vi "ConfigureDlg.vi"(8 "error in (no error)":errorcluster, 11 "Local in":refnum<class "Local.lvclass">) -> (0 "error out":errorcluster, 2 "Changed?":bool, 3 "Local out":refnum<class "Local.lvclass">)   [LabVIEW 2014, in "SyncPlugins.lvlib" / "Local.lvclass"]
uses:
  Local.lvclass
panel:
  in  "btnDone":bool
  # "Local Sync Module has no configurable Parameters"
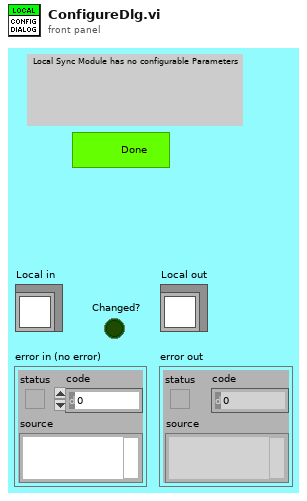
[diagram p1: front panel]
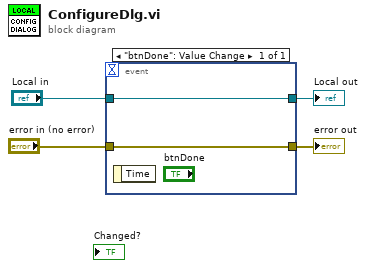
[diagram p0: block diagram]
diagram:
  n1 = event shown="[0] \"btnDone\": Value Change" {
    selector: _ -> [_]
    dyn-events: _ -> [_]
    timeout: _ -> [_]
    tunnel: "error in (no error)" -> [w6]
    tunnel: [w6] -> w3
    tunnel: [w5] -> w1
    tunnel: "Local in" -> [w5]
    event "btnDone": Value Change {
      n2 = event-data() -> ()  [unwired: 1 in, 1 out]
    }
  }
  "error out" <- w3
  "Local out" <- w1
